vi "ExpAvAt.vi"() -> ()   [LabVIEW 2011]
uses:
  <vilib>/Simulation/Scripting/Companion Diagram/SimConfigNode/SimParams.ctl
  <vilib>/Simulation/Scripting/Companion Diagram/SimConfigNode/_simSolvers.ctl
  <vilib>/Simulation/Implementation/Shared/SIMSCR Execution Mode.ctl
  <vilib>/Platform/TimedLoop/XDataNode/timing_clust.ctl
  <vilib>/Platform/TimedLoop/XDataNode/nitl_modes.ctl
  <vilib>/Platform/TimedLoop/XDataNode/wakeup.ctl
  <vilib>/Simulation/Param Hierarchy/Typedefs/SIMPH Param Control Actions.ctl
  <vilib>/Simulation/Scripting/Editor Utilities/SIM subVI tag data.ctl
  <vilib>/Simulation/Scripting/Editor Utilities/SIM subVI execution type.ctl
  <vilib>/Simulation/Implementation/Shared/NILVSim_FinishedLate.vi
  <vilib>/Simulation/Nonlinear/Implementation/NILVSim Saturation.llb/SIM Saturation (scalar).vi
  <vilib>/Simulation/SignalArithmetic/Implementation/NILVSim Gain.llb/SIM Gain (scalar).vi
  <vilib>/Simulation/Utility/Implementation/SIM Halt.vi
  <vilib>/Simulation/ContinuousLinear/Implementation/NILVSim ZeroPoleGain Direct.llb/SIM  ZeroPoleGain Direct (SISO).vi
  <vilib>/Simulation/Implementation/Shared/SIM Fire Discrete SubVI.vi
  <vilib>/Simulation/Implementation/Shared/NILVSim_Manager.vi
  <vilib>/Simulation/Implementation/Shared/NILVSim_ParamChanged.vi
  <vilib>/Simulation/Implementation/Shared/NILVSim_FinalizeModel.vi
  <vilib>/Simulation/Implementation/Shared/SIM Fire Discrete SubVI (Core).vi
  <vilib>/Simulation/Implementation/Shared/SIM Unbundle Sim Info.vi
  <vilib>/Simulation/Implementation/Shared/NILVSim_GetModelError.vi
  <vilib>/Simulation/Implementation/Shared/SIM Bundle Sim Info.vi
  <vilib>/Simulation/Implementation/Shared/NILVSim_Initialize.vi
  Instance          13 12Saved   Exp9 .vi
  <vilib>/Simulation/Scripting/Companion Diagram/SimConfigNode/SimDog.xnode
  <vilib>/Platform/TimedLoop/XDataNode/XDataNode.xnode
  <vilib>/Simulation/Implementation/XNodeFramework/SimXNode/SimX.xnode
  Instance           8 12Saved   Exp9 .vi
  Instance           9 12Saved   Exp9 .vi
  Instance          10 12Saved   Exp9 .vi
  Instance          11 12Saved   Exp9 .vi
  Instance          12 12Saved   Exp9 .vi
  <vilib>/Platform/TimedLoop/XDataNode/XDNodeRunTimeDep.lvlib
  <vilib>/Simulation/Implementation/Shared/NI_SIM_Implementation.lvlib
panel:
  in  "Configurações\ndo controlador":cluster{"Kc":dbl, "Ti":dbl, "Td":dbl}
  in  "stop":bool
  in  "AO0 (auto)":T1={"Magnitude"=8.0, "Frequência"=0.01, "Offset"=0.0}
  in  "Set-point:\nMan / Auto":bool
  out "Medidas":dbl[][](graph)
  in  "AO0\n(manual)":dbl(slide) scale=-10.0..10.0
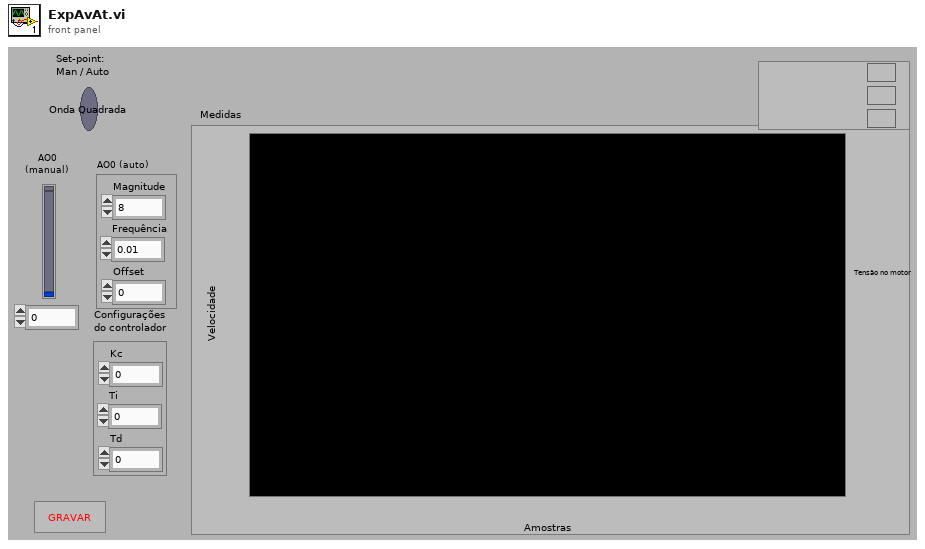
[diagram p1: front panel]
types:
  T1 = cluster{"Magnitude":dbl, "Frequência":dbl, "Offset":dbl}
  T2 = typedef "SIMPH Param Control Actions.ctl" = enum16{"get params", "set params"}
  T3 = typedef "SIM subVI tag data.ctl" = cluster{"period":dbl, "skew":dbl, "Simulation execution type":T4}
  T4 = typedef "SIM subVI execution type.ctl" = enum16{"Function call", "Discrete", "Continuous", "Initialization only", "Final step only"}
  T5 = typedef "XDNodeRunTimeDep.lvlib/timing_clust.ctl" = cluster{"Expected End [f-1]":u64, "Actual End [f-1]":u64, "Finished Late? [f-1]":bool, "Expected End [i-1]":u64, "Actual End [i-1]":u64, "Finished Late? [i-1]":bool, "Expected Start [i]":u64, "Actual Start [i]":u64, "Expected Start [f]":u64, "Actual Start [f]":u64, "Source Name":string, "Structure Name":string, "Period":i64, "Deadline":i64, "Offset":i64, "Start":i64, "Priority":i32, "Timeout":i32, "Mode":T6, "Wakeup Reason":T7, "Error":errorcluster, "Source Type":string, "Secondary Source Type":string, "Global End Time":u64, "Global Start Time":u64, "Frame Duration":u64, "Iteration Duration":u64, "Assigned CPU":i32, "I/O Scan Engine Mode":u32}
  T6 = typedef "XDNodeRunTimeDep.lvlib/nitl_modes.ctl" = enum32{"No Change", "Process missed periods, maintain original phase", "Discard missed periods, maintain original phase", "Process missed periods, ignore original phase", "Discard missed periods, ignore original phase"}
  T7 = typedef "XDNodeRunTimeDep.lvlib/wakeup.ctl" = enum32{"Normal", "Aborted", "Asynchronous wakeup", "Timing source error", "Timed loop error", "Timeout"}
  T8 = typedef "SimParams.ctl" = cluster{"Initial Time (s)":dbl, "Final Time (s)":dbl, "Step Size (s)":dbl, "ODE Solver":T9, "Minimum Step Size (s)":dbl, "Maximum Step Size (s)":dbl, "Relative Tolerance":dbl, "Absolute Tolerance":dbl, "Software Timing":bool, "Initial Step Size (s)":dbl, "Automatic Fixed Step Size?":bool, "Automatic Discrete Step Size?":bool, "Discrete Step Size (s)":dbl, "Calculate using Time Step":bool, "Solver Wired?":bool, "Prev.Frm.Expected End":u64, "Prev.Frm.Actual End":u64, "Prev.Frm.Finished Late?":bool, "Prev.Iter.Expected End":u64, "Prev.Iter.Actual End":u64, "Prev.Iter.Finished Late?":bool, "Expected Iteration Start":u64, "Actual Iteration Start":u64, "Expected Frame Start":u64, "Actual Frame Start":u64, "Source Name":string, "Name":string, "Period":i64, "Deadline":i64, "Offset":i64, "Start":i64, "Priority":i32, "Timeout":i32, "Processor":i32, "Mode":enum32{"No Change", "Process missed periods, maintain original phase", "Discard missed periods, maintain original phase", "Process missed periods, ignore original phase", "Discard missed periods, ignore original phase"}, "Wakeup reason":enum32{"Normal", "Aborted", "Asynchronous wakeup", "Timing source error", "Timed loop error", "Timeout"}, "Error":errorcluster, "Source Type":string, "Secondary Source Type":string, "Global End Time":u64, "Global Start Time":u64, "Full Solver Reset":bool, "Execution Mode":T10, "Nan/Inf Check":bool, "Custom Solver Library":string, "Solver Is Variable":bool, "custom solver name":string}
  T9 = typedef "_simSolvers.ctl" = enum16{"Runge-Kutta 1 (Euler)", "Runge-Kutta 2", "Runge-Kutta 3", "Runge-Kutta 4", "Runge-Kutta 23 (variable)", "Runge-Kutta 45 (variable)", "BDF (variable)", "Adams-Moulton (variable)", "Rosenbrock (variable)", "Discrete States Only", "Linearizer", "State Query", "Trim Eval", "Custom Solver"}
  T10 = typedef "SIMSCR Execution Mode.ctl" = u16
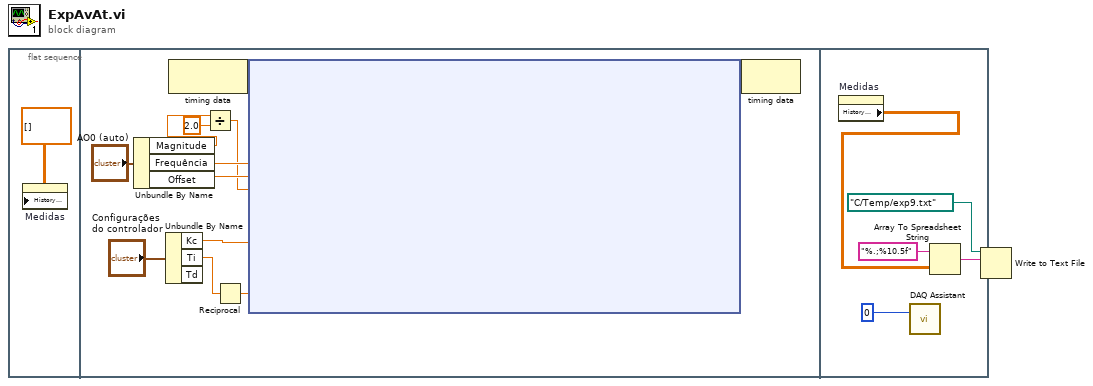
[diagram p0: block diagram]
diagram:
  n1 = flat-sequence {
    frame #0 {
      n2 = property on="Medidas" class="WFChart (strict)"("History Data"=dbl[][] []) -> ()  [unwired: 2 in, 2 out]
    }
    frame #1 {
      n3 = Unbundle By Name("AO0 (auto)") -> ("Magnitude"=w4:dbl, "Frequência"=w10:dbl, "Offset"=w9:dbl)
      n4 = Unbundle By Name("Configurações\ndo controlador") -> ("Kc"=w7:dbl, "Ti"=w5:dbl)  [unwired: 1 out]
      n5 = node-c288() -> (w13:variant)  [unwired: 1 in]
      n6 = Divide(x=w4, y=2.0) -> (x/y=w2:dbl)
      n7 = Reciprocal(x=w5) -> (1/x=w6:dbl)
      n8 = node-c254 ("Control & Simulation Loop")(w13, w10, w9, w7, w6, w2) -> (w12:variant)
      n9 = node-c288(w12) -> ()  [unwired: 1 out]
    }
    frame #2 {
      n10 = property on="Medidas" class="WFChart (strict)"() -> ("History Data"=w294:dbl[][])  [unwired: 2 in, 2 out]
      n11 = call "DAQ Assistant"("data"=0) -> ()  [unwired: 17 in, 2 out]
      n12 = Array To Spreadsheet String(array=w294, 3:"%.;%10.5f" ("format string")) -> (spreadsheet string=w297:string)  [unwired: 1 in]
      n13 = Write to Text File(file (use dialog)=path "C:/Temp/exp9.txt", text=w297) -> ()  [unwired: 2 in, 3 out]
    }
  }
